vi "timed_PRBS_MLS_bit_generator.vi"(10 "Bit Length\n(how long is the sequence)":i64, 11 "Bit Size (seconds per bit)":dbl) -> (1 "mls sequence":u8[](array[numeric]), 2 "Which Bit are we at?":dbl, 3 "simulation time":dbl, 4 "MLS PRBS output":u8)   [LabVIEW 2020]
uses:
  PRBS_bit_generator_indexer.vi
  <vilib>/Simulation/Implementation/Shared/SIMSCR Execution Mode.ctl
  <vilib>/Simulation/Scripting/Companion Diagram/SimConfigNode/SimParams.ctl
  <vilib>/Simulation/Scripting/Companion Diagram/SimConfigNode/_simSolvers.ctl
  <vilib>/Simulation/Param Hierarchy/Typedefs/SIMPH Param Control Actions.ctl
  <vilib>/Simulation/Implementation/Shared/NILVSim_ParamChanged.vi
  <vilib>/Simulation/Implementation/Shared/NILVSim_FinishedLate.vi
  <vilib>/Simulation/Implementation/Shared/NILVSIM_BeginStep.vi
  <vilib>/Simulation/Utility/Implementation/SIM Time.vi
  <vilib>/Simulation/Implementation/Shared/NILVSim_Manager.vi
  <vilib>/Utility/error.llb/Clear Errors.vi
  <vilib>/Simulation/Implementation/Shared/NILVSim_FinalizeModel.vi
  <vilib>/Simulation/Implementation/Shared/SIM Unbundle Sim Info.vi
  <vilib>/Simulation/Implementation/Shared/NILVSim_Initialize.vi
  <vilib>/Simulation/Utility/Implementation/NILVSim Get Time and IsAcceptedStep.vi
  <vilib>/Simulation/Implementation/Shared/NILVSim_GetModelError.vi
  <vilib>/Simulation/Implementation/Shared/SIM SimErrorHandler.vi
  <vilib>/Simulation/Implementation/Shared/SIMSH Read Queue.vi
  <vilib>/Simulation/Implementation/Shared/SIM Bundle Sim Info.vi
  <vilib>/Simulation/Scripting/Companion Diagram/SimConfigNode/SimDog.xnode
  <vilib>/Simulation/Implementation/XNodeFramework/SimXNode/SimX.xnode
  <vilib>/Simulation/Implementation/Shared/NI_SIM_Implementation.lvlib
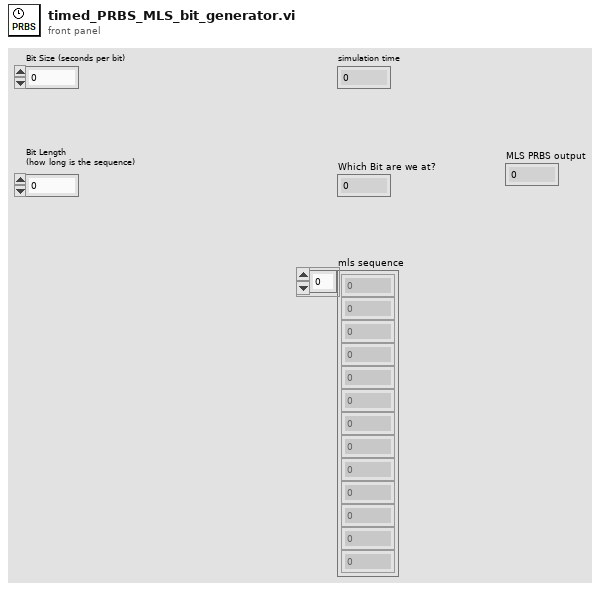
[diagram p1: front panel]
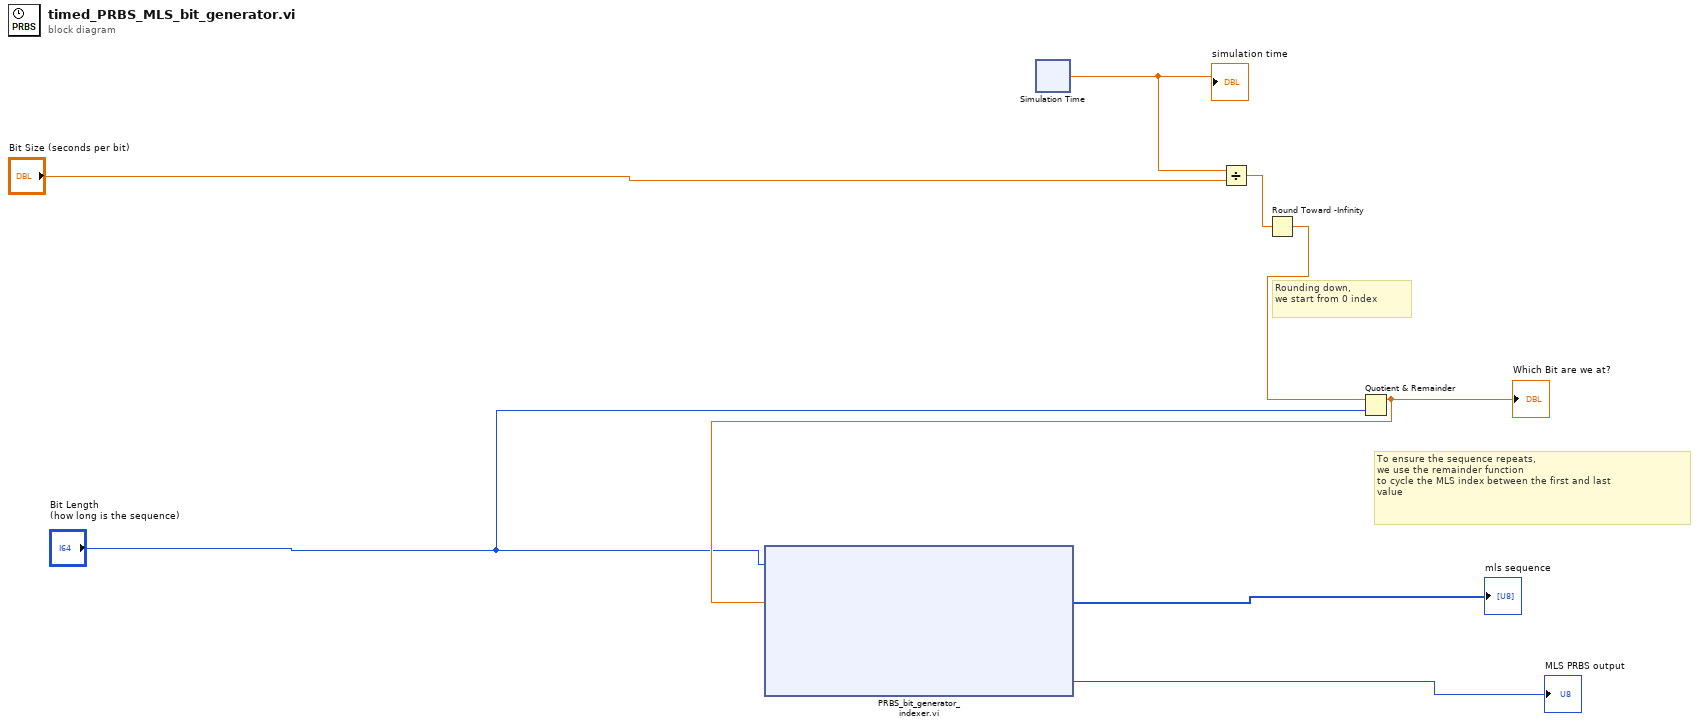
[diagram p0: block diagram]
diagram:
  # "To ensure the sequence repeats, \nwe use the remainder function\nto cycle the MLS index between the first and last \nvalue"
  # "Rounding down,\nwe start from 0 index"
  n1 = xnode "Simulation Time"() -> ("simulation time"=w1:dbl)  [unwired: 2 in]
  "simulation time" <- w1
  n2 = Divide(x=w1, y="Bit Size (seconds per bit)") -> (x/y=w6:dbl)
  n3 = Round Toward -Infinity(1:w6) -> (0:w4:dbl)
  n4 = Quotient & Remainder(x=w4, y="Bit Length\n(how long is the sequence)") -> (x-y*floor(x/y)=w8:dbl)  [unwired: 1 out]
  "Which Bit are we at?" <- w8
  n5 = xnode "PRBS_bit_generator_indexer.vi"("MLS array index\n\nNote: start from 0"=w8, "Bit Length\n(how many bits does the sequence have)"="Bit Length\n(how long is the sequence)") -> ("mls sequence"=→"mls sequence":u8[], "MLS output"=→"MLS PRBS output":u8)  [unwired: 8 out]
